vi "startEvent.vi"(8 "error in (no error)":errorcluster, 11 "ExperimentControl in":refnum<class "ExperimentControl.lvclass">) -> (0 "error out":errorcluster, 3 "ExperimentControl out":refnum<class "ExperimentControl.lvclass">)   [LabVIEW 2011, in "Views.lvlib" / "ExperimentControl.lvlib" / "ExperimentControl.lvclass"]
uses:
  ExperimentControl.lvclass
  ExperimentControl.lvclass/ExperimentControl.ctl
  Hal/HWController/HWControllerEvents/HWControllerEvents.lvclass
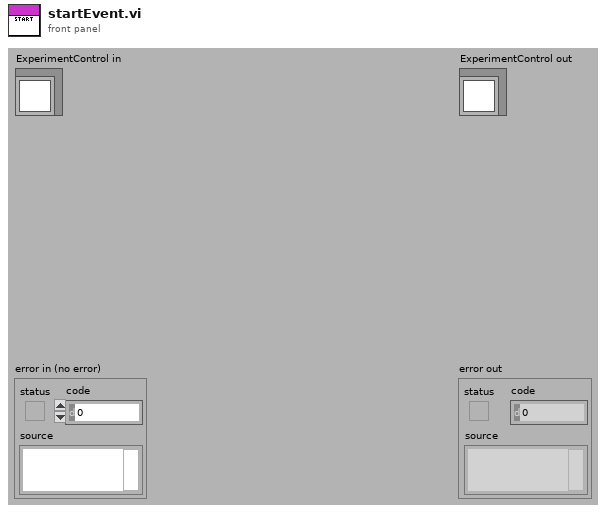
[diagram p1: front panel]
types:
  T1 = enum16{"start", "stop", "statusInquiry", "configure", "resetError", "resourcesInquiry", "reserveResources", "initialise", "resetAllChannels", "staticUpdate", "close", "HWStatus", "error", "resourcesAvailable", "resourcesReserved", "compilerError", "compiledScript", "compilingScript", "runScript", "configureCompiledScript"}
  T2 = cluster{"incomingEventTypes":cluster{"start":cluster{"Boolean":bool}, "stop":cluster{"Boolean":bool}, "statusInquiry":cluster{"Boolean":bool}, "configure":cluster{"DPScriptPath":path, "TimeStamp":string, "HWLoop?":bool}, "resetError":cluster{"Boolean":bool}, "resourcesInquiry":cluster{"Boolean":bool}, "reserveResources":cluster{"HWList":string[]}, "initialise":cluster{"HWList":string[]}, "close":cluster{"Boolean":bool}, "resetAllChannels":cluster{"Boolean":bool}, "staticChannelUpdate":cluster{"channel_address":string, "calibratedValue":dbl}, "runScript":cluster{"DPScriptPath":path, "TimeStamp":string, "HWLoop?":bool}, "compilingScript":cluster{"Path":path}, "compiledScript":cluster{"Path":path, "timeCompileAt":string}, "compilerError":cluster{"Path":path}, "configureCompiledScript":cluster{"DPScriptPath":path, "TimeStamp":string, "HWLoop?":bool, "CompiledScript":cluster{"ScriptListCompiler.lvclass":refnum<class "ScriptListCompiler.lvclass">, "aoChannels":refnum<class "AnalogOutput.lvclass">[], "doChannels":refnum<class "DigitalOutput.lvclass">[], "rfChannels":refnum<class "DDSOutput.lvclass">[]}}, "restartCompiler":cluster{"restart":bool}, "staticRfChannelUpdate":cluster{"channel_address":string, "Output":cluster{"Frequency(MHz)":dbl, "Amplitude":dbl, "Phase":dbl, "OutputForm":enum16{"Sine", "Square", "Triangle", "Arbitrary"}}}, "cameraUpdate":cluster{"Camera":string, "Type":string, "settings":path}}, "outgoingEventTypes":cluster{"HWStatus":cluster{"status":enum16{"Ready", "Compiling", "Configured", "Running", "Stopping", "Unresolved Error"}}, "error":cluster{"error out":errorcluster}, "resourcesAvailable":cluster{"availableHWList":string[], "reservedHWList":string[]}, "resourcesReserved":cluster{"reservedHWList":string[]}}}
  T3 = cluster{"eventId":enum16{"start", "stop", "statusInquiry", "configure", "resetError", "resourcesInquiry", "reserveResources", "initialise", "resetAllChannels", "staticUpdate", "close", "HWStatus", "error", "resourcesAvailable", "resourcesReserved", "compilerError", "compiledScript", "compilingScript", "runScript", "configureCompiledScript"}, "start":cluster{"Boolean":bool}}
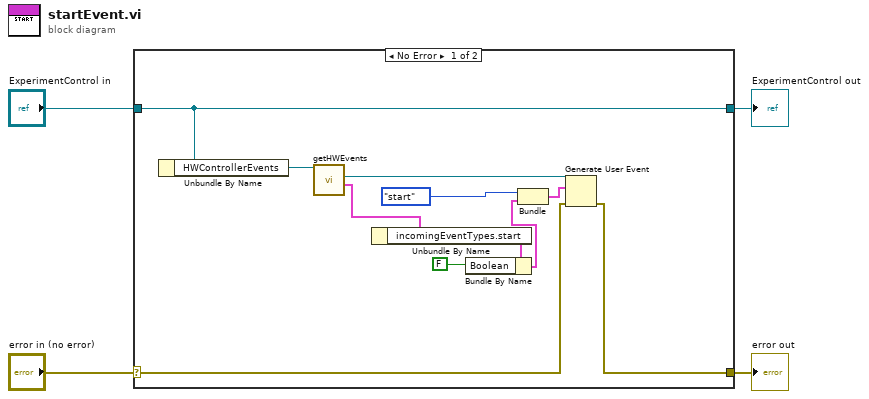
[diagram p0: block diagram]
diagram:
  n1 = case shown="No Error" "error in (no error)" {
    selector: "error in (no error)" -> [w5 w17]
    tunnel: [w6 w17] -> w3
    tunnel: [w15 w16] -> w1
    tunnel: "ExperimentControl in" -> [w15 w16]
    frame No Error {
      n2 = Unbundle By Name(w15) -> ("HWControllerEvents"=w14:refnum<class "HWControllerEvents.lvclass">)
      n3 = call-dynamic "getHWEvents.vi"("HWControllerEvents in"=w14) -> ("eventDataTypes"=w7:T2, "HWCEvent"=w8:refnum<user-event>)  [unwired: 7 in, 2 out]
      n4 = Unbundle By Name(w7) -> ("incomingEventTypes.start"=w12:cluster{"Boolean":bool})
      n5 = Bundle By Name(cluster=w12, "Boolean"=FALSE) -> (w11:cluster{"Boolean":bool})
      n6 = Bundle("eventId"=T1."start", "start"=w11) -> (w13:T3)  [unwired: 1 in]
      n7 = Generate User Event(user event=w8, event data cluster=w13, error in=w5) -> (error out=w6:errorcluster)  [unwired: 1 out]
    }
    frame Error {
    }
  }
  "error out" <- w3
  "ExperimentControl out" <- w1
